vi "Harmonics MSMT Set Signal Name.vi"(8 "error in (no error)":errorcluster, 9 "Harmonic Order":i8, 10 "Step In":refnum<k7>, 11 "Harmonics in":refnum<class "Harmonics.lvclass">) -> (0 "error out":errorcluster, 2 "Step Out":refnum<k7>, 3 "Harmonics out":refnum<class "Harmonics.lvclass">)   [LabVIEW 2018, in "Harmonics.lvlib" / "Harmonics.lvclass"]
uses:
  Harmonics.lvclass
  C:/Sequence Automation/Plugins/Measurement Interface.lvlibp/Measurement Interface.lvclass
  Plugins/Measurement Interface.lvlibp/Private Methods/Measurement Parameters/Read Measurement Parameters.vi
  Plugins/String Database.lvlibp/String Database.lvclass
  Plugins/TestStand API Tools (TSAT).lvlibp/Step Actions/TSAT Step Actions.lvlib
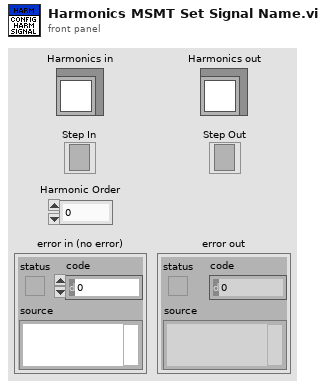
[diagram p1: front panel]
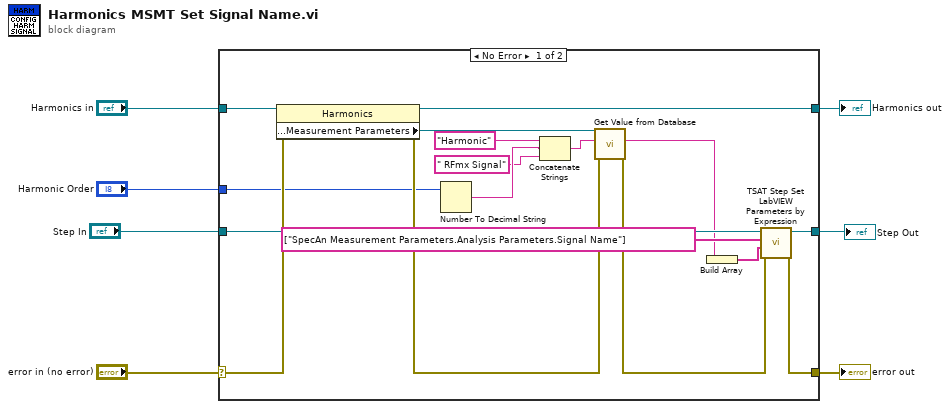
[diagram p0: block diagram]
diagram:
  n1 = case shown="No Error" "error in (no error)" {
    selector: "error in (no error)" -> [w24 w27]
    tunnel: [w14 w27] -> w6
    tunnel: [w22 w26] -> w4
    tunnel: "Harmonics in" -> [w23 w26]
    tunnel: "Harmonic Order" -> [w18 _]
    tunnel: [w17 w25] -> w2
    tunnel: "Step In" -> [w16 w25]
    frame No Error {
      n2 = property class="Harmonics"(reference=w23, error in=w24) -> (reference out=w22:refnum<class "Harmonics.lvclass">, error out=w19:errorcluster, "Protected Methods:Measurement Parameters"=w21:refnum<class "String Database.lvclass">)
      n3 = Number To Decimal String(number=w18) -> (decimal integer string=w11:string)  [unwired: 1 in]
      n4 = Concatenate Strings("Harmonic" ("Entry Name"), w11, " RFmx Signal" ("string")) -> (w12:string)
      n5 = call "Get Value from Database.vi"("error in (no error)"=w19, "Entry Name"=w12, "Message in"=w21) -> ("error out"=w15:errorcluster, "Entry Value"=w9:string)  [unwired: 5 in, 2 out]
      n6 = Build Array(w9) -> (w8:string[])
      n7 = call "TSAT Step Set LabVIEW Parameters by Expression.vi"("Error In"=w15, "Value Expressions"=w8, "Parameters to Set"=string[] ["SpecAn Measurement Parameters.Analysis Parameters.Signal Name"], "Step In"=w16) -> ("Error Out"=w14:errorcluster, "Step Out"=w17:refnum<k7>)  [unwired: 6 in]
    }
    frame Error {
    }
  }
  "error out" <- w6
  "Harmonics out" <- w4
  "Step Out" <- w2
